vi "init.vi"(8 "error in (no error)":errorcluster, 11 "PressureValveTC in":refnum<class "PressureValveTC.lvclass">) -> (0 "error out":errorcluster, 3 "PressureValveTC out":refnum<class "PressureValveTC.lvclass">)   [LabVIEW 2015, in "PressureValveTC.lvclass"]
uses:
  PressureValveTC.lvclass
  <userlib>/Common/Devices/PressureValve/PressureValve/PressureValve.lvclass
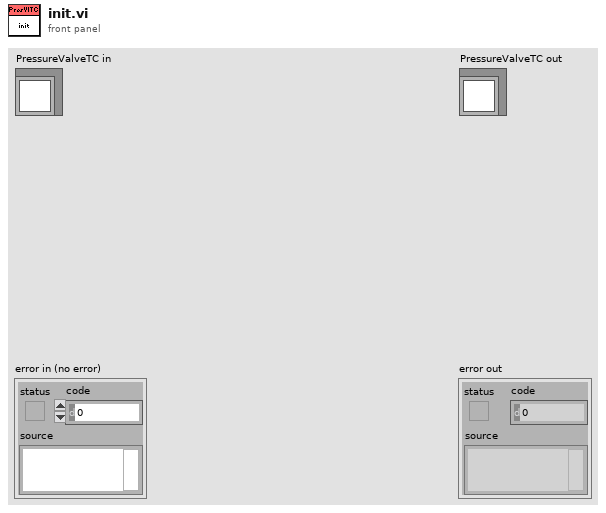
[diagram p1: front panel]
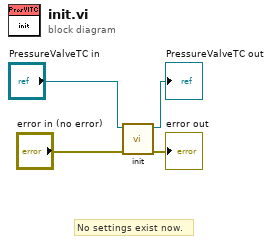
[diagram p0: block diagram]
diagram:
  # "No settings exist now."
  n1 = call-parent "init.vi"("error in (no error)"="error in (no error)", "PressureValve in"="PressureValveTC in") -> ("error out"=→"error out":errorcluster, "PressureValve out"=→"PressureValveTC out":refnum<class "PressureValveTC.lvclass">)  [unwired: 8 in]
